vi "CheckDoubleClick.vi"(8 "error in (no error)":errorcluster, 11 "cPass":bool) -> (0 "error out":errorcluster, 2 "Perform?":bool, 3 "Double Click?":bool)   [LabVIEW 2013]
doc: "Determines which pass method to use and whether to actually call the pass VI.\n\nAccepts the raw controller input (<B>cPass</B>).\nA <B>single</B> button press will select the <B>Ground Pass</B> (True).\nA <B>double</B> button press (i.e. double click) will select the <B>Elevated Pass</B> (False).\nAfter a small delay (250 ms), the VI will output True from <B>Perform?</B>, indicating input can be passed to the Toggle / Pass vi (in a nested case structure)."
uses:
  DoubleClickStates.ctl
panel:
  in  "Timeout":u32=250
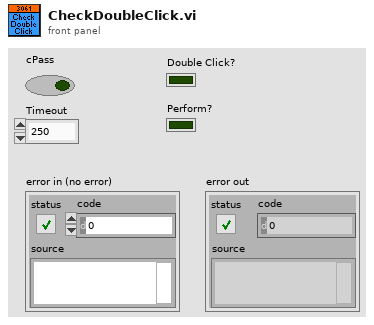
[diagram p1: front panel]
types:
  T1 = typedef "DoubleClickStates.ctl" = enum16{"WaitForClick", "WaitForDoubleClick", "SingleClick", "DoubleClick"}
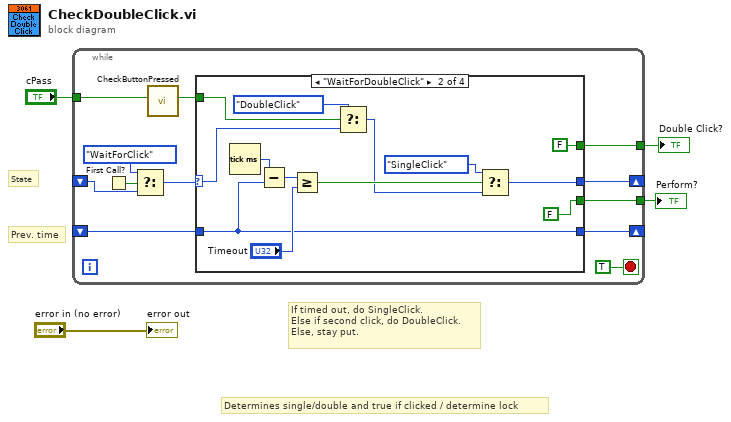
[diagram p0: block diagram]
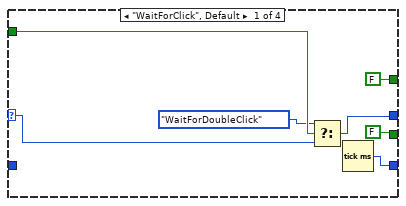
[diagram p2: hidden frame]
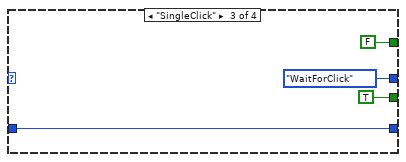
[diagram p3: hidden frame]
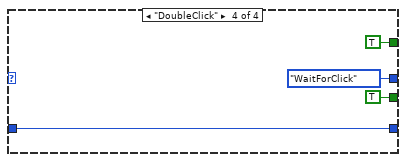
[diagram p4: hidden frame]
diagram:
  # "If timed out, do SingleClick.\nElse if second click, do DoubleClick.\nElse, stay put."
  # "Determines single/double and true if clicked / determine lock"
  # "Prev. time"
  # "State"
  n1 = while {
    shift-right: [w11] -> _
    shift-left: _ -> [w13]
    shift-right: [w10] -> _
    shift-left: _ -> [w9]
    tunnel: "cPass" -> [w6]
    tunnel: [w8] -> w2
    tunnel: [w7] -> w1
    stop <- TRUE stop-if-true
    n2 = First Call?() -> (First Call?: T/F=w15:bool)
    n3 = Select(t=DoubleClickStates."WaitForClick", s=w15, f=w13) -> (s? t:f=w12:T1)
    n4 = call "CheckButtonPressed.vi"("Button"=w6) -> ("Pressed?"=w5:bool)  [unwired: 9 in, 1 out]
    n5 = case shown="\"WaitForDoubleClick\"" w12 {
      selector: w12 -> [w17 w28 _ _]
      tunnel: [w23 w26 DoubleClickStates."WaitForClick" DoubleClickStates."WaitForClick"] -> w11
      tunnel: [w22 w24 w38 w43] -> w10
      tunnel: w9 -> [_ w24 w38 w43]
      tunnel: [FALSE FALSE TRUE TRUE] -> w8
      tunnel: [FALSE FALSE FALSE TRUE] -> w7
      tunnel: w5 -> [w20 w30 _ _]
      frame "WaitForClick", Default {
        n6 = Select(t=DoubleClickStates."WaitForDoubleClick" ("f"), s=w20, f=w17) -> (s? t:f=w23:T1)
        n7 = Tick Count (ms)() -> (millisecond timer value=w22:u32)
      }
      frame "WaitForDoubleClick" {
        n8 = Tick Count (ms)() -> (millisecond timer value=w32:u32)
        n9 = Subtract(x=w32, y=w24) -> (x-y=w36:u32)
        n10 = Greater Or Equal?(x=w36, y="Timeout") -> (x >= y?=w35:bool)
        n11 = Select(t=DoubleClickStates."DoubleClick", s=w30, f=w28) -> (s? t:f=w27:T1)
        n12 = Select(t=DoubleClickStates."SingleClick", s=w35, f=w27) -> (s? t:f=w26:T1)
      }
      frame "SingleClick" {
      }
      frame "DoubleClick" {
      }
    }
  }
  "Perform?" <- w2
  "Double Click?" <- w1
  "error out" <- "error in (no error)"
